vi "GSW.vi"() -> ()   [LabVIEW 2019]
panel:
  in  "Path to Code":path
  # "A lot of links here"
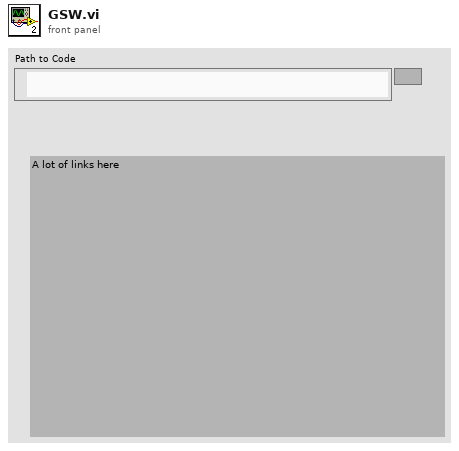
[diagram p1: front panel]
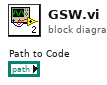
[diagram p0: block diagram]
diagram:
